vi "Test Subscriber.vi"() -> ()   [LabVIEW 2021]
uses:
  ChannelCommon/typedef/Datatype Waveform.ctl
  CIFChannels/Typedef/Direction.ctl
  CIF_NIChn_FIFO_DAQ.lvclass
  CIFChannels/CIFChannels.lvclass
  ChannelCommon/ChannelCommon.lvlib
panel:
  in  "stop":bool
  out "timed out?":bool
  out "DAQ Out":T1[](array[typedef])
  out "error out":errorcluster
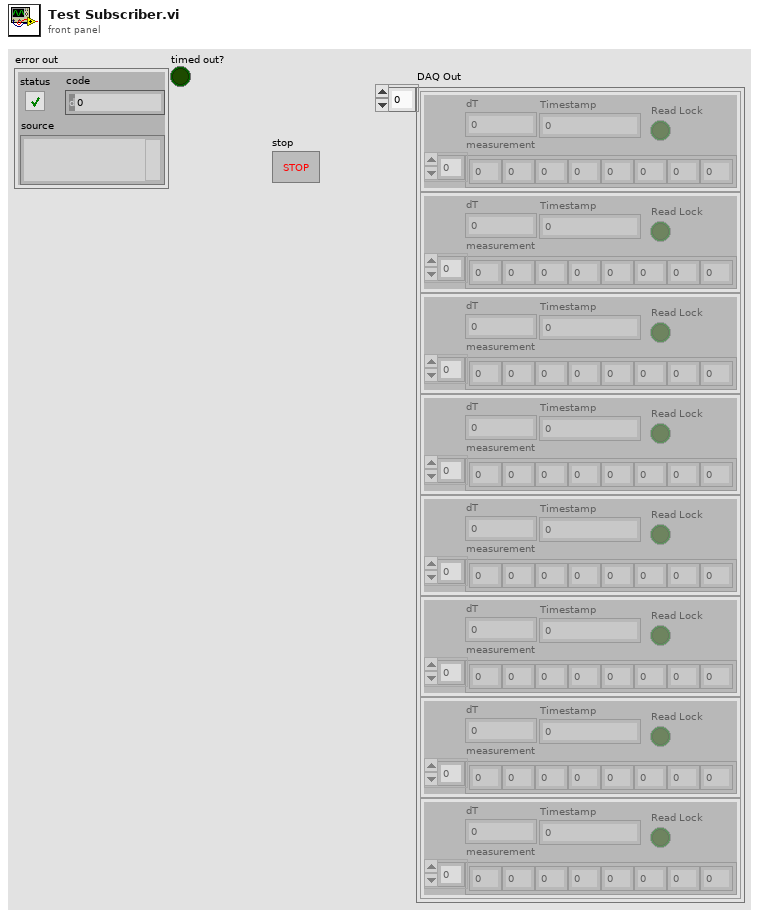
[diagram p1: front panel]
types:
  T1 = typedef "ChannelCommon.lvlib/Datatype Waveform.ctl" = cluster{"measurement":dbl[], "dT":dbl, "Timestamp":i64, "Read Lock":bool}
  T2 = typedef "CIFChannels.lvclass/Direction.ctl" = enum16{"Publisher", "Subscriber"}
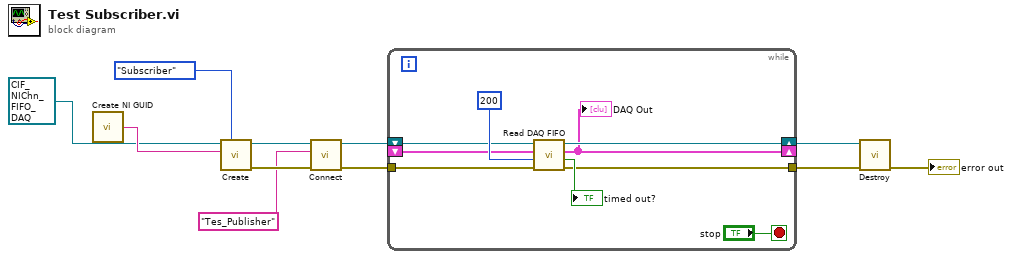
[diagram p0: block diagram]
diagram:
  n1 = call <vilib>:"Create NI GUID.vi"() -> ("NI GUID"=w7:string)
  n2 = call-dynamic "Create.vi"("Direction"=Direction."Subscriber", "Name"=w7, "CIFFIFO in"=refnum<class "CIF_NIChn_FIFO_DAQ.lvclass"> refnum ("CIF_NIChn_FIFO_DAQ.lvclass")) -> ("error out"=w8:errorcluster, "CIFFIFO out"=w9:refnum<class "CIF_NIChn_FIFO_DAQ.lvclass">)  [unwired: 7 in]
  n3 = call-dynamic "Connect.vi"("error in (no error)"=w8, "Connection Name"="Tes_Publisher", "CIFTag in"=w9) -> ("error out"=w3:errorcluster, "CIFTag out"=w6:refnum<class "CIF_NIChn_FIFO_DAQ.lvclass">)  [unwired: 7 in]
  n4 = while {
    shift-right: [w20] -> w11
    shift-left: w6 -> [w18]
    tunnel: w3 -> [w17]
    tunnel: [w15] -> w2
    shift-right: [w13] -> _
    shift-left: _ -> [w12]
    stop <- "stop" stop-if-true
    n5 = call-dynamic "Read DAQ FIFO.vi"("error in (no error)"=w17, "Timeout (ms)"=200, "Data In"=w12, "CIF_NIChn_FIFO_DAQ in"=w18) -> ("error out"=w15:errorcluster, "timed out?"=→"timed out?":bool, "Data Out"=w13:T1[], "CIF_NIChn_FIFO_DAQ out"=w20:refnum<class "CIF_NIChn_FIFO_DAQ.lvclass">)  [unwired: 3 in, 1 out]
    "DAQ Out" <- w13
  }
  n6 = call-dynamic "Destroy.vi"("error in (no error)"=w2, "CIFFIFO in"=w11) -> ("error out"=→"error out":errorcluster)  [unwired: 8 in, 1 out]
